vi "Temproray.vi"(11 "Options in":refnum<class "Options.lvclass">) -> (3 "Options out":refnum<class "Options.lvclass">)   [LabVIEW 2020, in "Approval Tests.lvlib"]
uses:
  Approval Tests.lvlib
  Options/Options.lvclass
  Options/Options.lvclass/Options.ctl
  Naming Data/Naming Data.lvclass/Naming Data.ctl
  Options/Read Naming Data.vi
  Naming Data/Read Test VI Name.vi
  Naming Data/Write Test VI Name.vi
  Options/Write Naming Data.vi
  Naming Data/Naming Data.lvclass
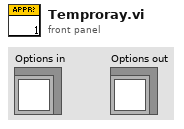
[diagram p1: front panel]
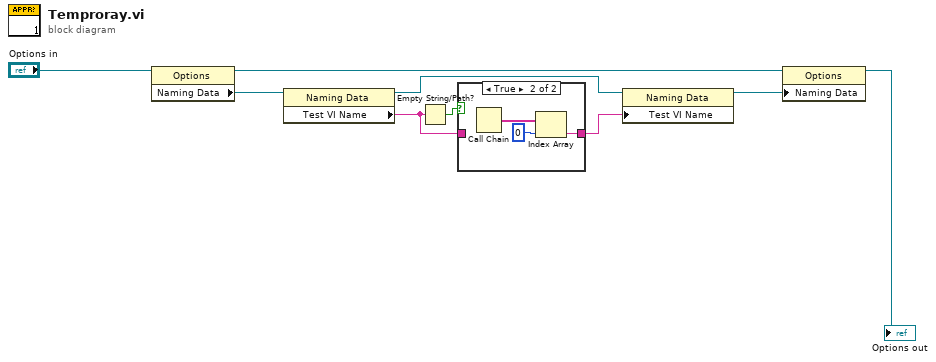
[diagram p0: block diagram]
diagram:
  n1 = property class="Options"(reference="Options in") -> (reference out=w6:refnum<class "Options.lvclass">, "Naming Data"=w2:refnum<class "Naming Data.lvclass">)  [unwired: 1 in, 1 out]
  n2 = property class="Naming Data"(reference=w2) -> (reference out=w3:refnum<class "Naming Data.lvclass">, "Test VI Name"=w4:string)  [unwired: 1 in, 1 out]
  n3 = Empty String/Path?(string/path=w4) -> (empty?=w1:bool)
  n4 = case shown="True" w1 {
    tunnel: w4 -> [w10 _]
    tunnel: [w10 w13] -> w5
    frame False {
    }
    frame True {
      n5 = Call Chain() -> (call chain=w11:string[])
      n6 = Index Array(array=w11, index=0) -> (element=w13:string)
    }
  }
  n7 = property class="Naming Data"(reference=w3, "Test VI Name"=w5) -> (reference out=w8:refnum<class "Naming Data.lvclass">)  [unwired: 1 in, 1 out]
  n8 = property class="Options"(reference=w6, "Naming Data"=w8) -> (reference out=→"Options out":refnum<class "Options.lvclass">)  [unwired: 1 in, 1 out]
